vi "SH_NumberOfShapelets.vi"(8 "error in (no error)":errorcluster, 9 "MaxLength (in %)":dbl(slide) min=0.0 max=1.0 step=0.05 scale=0.0..1.0, 10 "MinLength (in %)":dbl(slide) min=0.0 max=1.0 step=0.05 scale=0.0..1.0, 11 "ShapeletClass in":refnum<class "Shapelets Search Brute Force.lvclass">) -> (0 "error out":errorcluster, 2 "Number of Shapelets":i32, 3 "ShapeletClass out":refnum<class "Shapelets Search Brute Force.lvclass">)   [LabVIEW 2016, in "Shapelets Search (Brute Force).lvlib" / "Shapelets Search Brute Force.lvclass"]
uses:
  Shapelets Search Brute Force.lvclass
  Shapelets Search Brute Force.lvclass/Shapelets Search Brute Force.ctl
panel:
  # "This VI is a part of BCI Design library, http://www.ru-bci.org \nCopyright © 2020, Sotnikov Peter, All rights reserved. License: CC BY-NC 4.0"
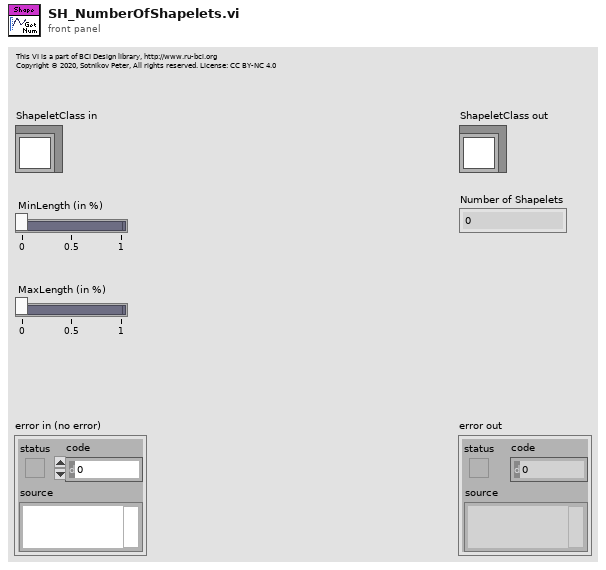
[diagram p1: front panel]
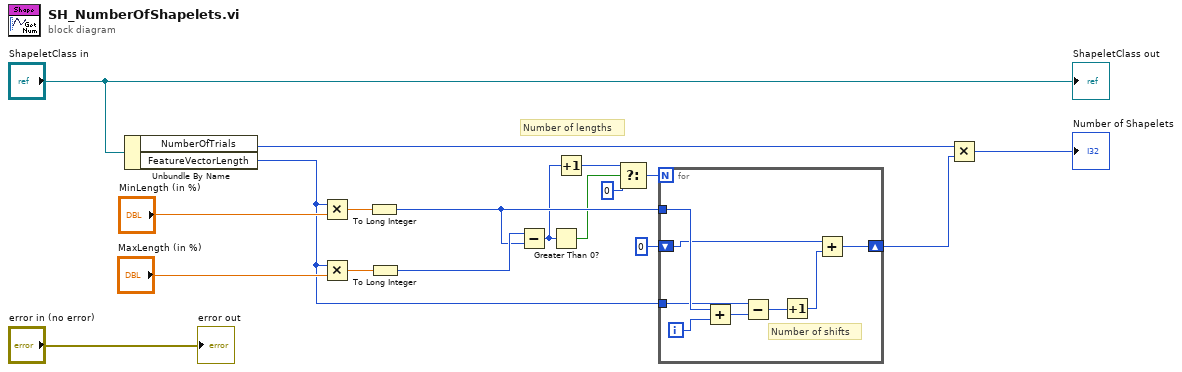
[diagram p0: block diagram]
diagram:
  # "Number of lengths"
  n1 = Unbundle By Name("ShapeletClass in") -> ("NumberOfTrials"=w9:i32, "FeatureVectorLength"=w1:i32)
  n2 = Multiply(x=w1, y="MinLength (in %)") -> (x*y=w15:dbl)
  n3 = Multiply(x=w1, y="MaxLength (in %)") -> (x*y=w13:dbl)
  n4 = To Long Integer(number=w15) -> (32bit integer=w11:i32)
  n5 = To Long Integer(number=w13) -> (32bit integer=w12:i32)
  n6 = Subtract(x=w12, y=w11) -> (x-y=w5:i32)
  n7 = Greater Than 0?(x=w5) -> (x > 0?=w6:bool)
  n8 = Increment(x=w5) -> (x+1=w4:i32)
  n9 = Select(t=w4, s=w6, f=0) -> (s? t:f=w3:i32)
  n10 = for {
    N: w3 -> [_]
    tunnel: w11 -> [w25]
    tunnel: w1 -> [w24]
    shift-right: [w22] -> w8
    shift-left: 0 -> [w21]
    i -> [w26]
    # "Number of shifts"
    n11 = Add(x=w25, y=w26) -> (x+y=w23:i32)
    n12 = Subtract(x=w24, y=w23) -> (x-y=w20:i32)
    n13 = Increment(x=w20) -> (x+1=w19:i32)
    n14 = Add(x=w21, y=w19) -> (x+y=w22:i32)
  }
  n15 = Multiply(x=w9, y=w8) -> (x*y=→"Number of Shapelets":i32)
  "error out" <- "error in (no error)"
  "ShapeletClass out" <- "ShapeletClass in"
